vi "Set Active Controller on Name.vi"(8 "error in":errorcluster, 10 "Name":string, 11 "AC Comm in":refnum<class "AlicatCommBank.lvclass">) -> (0 "error out":errorcluster, 3 "AC Comm out":refnum<class "AlicatCommBank.lvclass">)   [LabVIEW 2015, in "Alicat.lvlib" / "AlicatCommBank.lvclass"]
uses:
  AlicatCommBank.lvclass
  Get Addresses.vi
  Get Dev Names.vi
  Write actCtl.vi
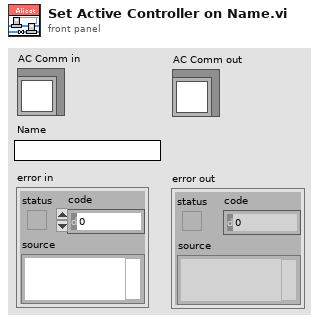
[diagram p1: front panel]
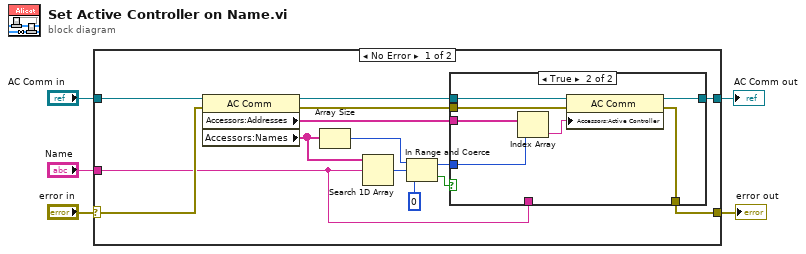
[diagram p0: block diagram]
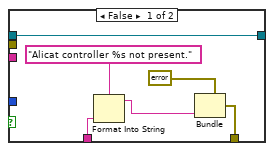
[diagram p2: hidden frame]
diagram:
  n1 = case shown="No Error" "error in" {
    selector: "error in" -> [w9 w34]
    tunnel: [w10 w34] -> w4
    tunnel: [w12 w33] -> w2
    tunnel: "AC Comm in" -> [w19 w33]
    tunnel: "Name" -> [w7 _]
    frame No Error {
      n2 = property class="AC Comm"(reference=w19, error in=w9) -> (reference out=w13:refnum<class "AlicatCommBank.lvclass">, error out=w11:errorcluster, "Accessors:Addresses"=w14:string[], "Accessors:Names"=w17:string[])
      n3 = Array Size(array=w17) -> (size(s)=w6:i32)
      n4 = Search 1D Array(1D array=w17, element=w7) -> (index of element=w18:i32)  [unwired: 1 in]
      n5 = In Range and Coerce(upper limit=w6, x=w18, lower limit=0) -> (coerced(x)=w15:i32, In Range?=w8:bool)
      n6 = case shown="True" w8 {
        tunnel: w15 -> [_ w32]
        tunnel: w14 -> [_ w31]
        tunnel: w13 -> [w25 w30]
        tunnel: [w25 w28] -> w12
        tunnel: w11 -> [_ w27]
        tunnel: [w21 w26] -> w10
        tunnel: w7 -> [w22 _]
        frame False {
          n7 = Format Into String(format string="Alicat controller %s not present.", w22) -> (resulting string=w20:string)  [unwired: 2 in, 1 out]
          n8 = Bundle(cluster=errorcluster {"status"=TRUE, "code"=-8000, "source"=""} ("error out"), "source"=w20) -> (w21:errorcluster)  [unwired: 2 in]
        }
        frame True {
          n9 = Index Array(array=w31, index=w32) -> (element=w29:string)
          n10 = property class="AC Comm"(reference=w30, error in=w27, "Accessors:Active Controller"=w29) -> (reference out=w28:refnum<class "AlicatCommBank.lvclass">, error out=w26:errorcluster)
        }
      }
    }
    frame Error {
    }
  }
  "error out" <- w4
  "AC Comm out" <- w2
